vi "IP Address Validity Check.vi"(11 "IP Address":string="192.168.1.2") -> (3 "IP Address Vaidity Check":bool)   [LabVIEW 2021, in "Modbus Master System Explorer.lvlib"]
uses:
  Modbus Master System Explorer.lvlib
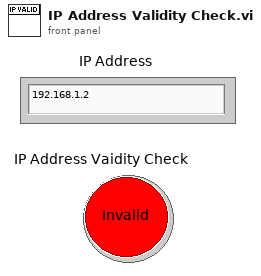
[diagram p1: front panel]
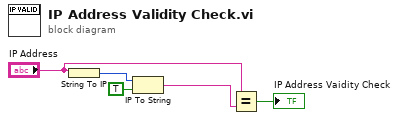
[diagram p0: block diagram]
diagram:
  n1 = String To IP(1:"IP Address") -> (0:w5:u32)
  n2 = IP To String(1:TRUE ("dot notation? (F)"), 2:w5) -> (0:w3:string)
  n3 = Equal?(x="IP Address", y=w3) -> (x = y?=→"IP Address Vaidity Check":bool)
